vi "detectISOSPIdebug.vi"(8 "errin":errorcluster) -> ()   [LabVIEW 2020]
uses:
  <vilib>/Instr/_visa.llb/VISA Find Search Mode.ctl
  <vilib>/Instr/_visa.llb/VISA Configure Serial Port (Instr).vi
panel:
  out "liste trouvée":string[](array[string])
  out "tableau ajouté":errorcluster[](array[cluster])
  out "Booléen":bool
  out "buffer de lecture":string
  # "2A49 444E 3F0A"
  # "*IDN?"
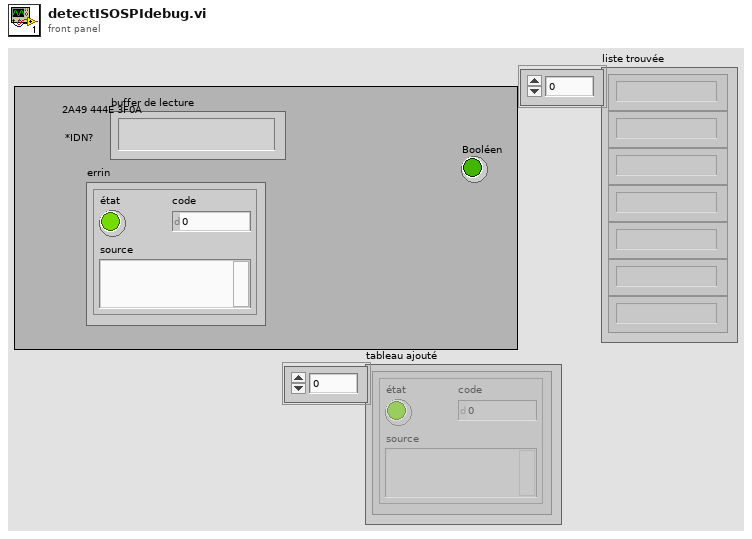
[diagram p1: front panel]
types:
  T1 = typedef "VISA Find Search Mode.ctl" = u32
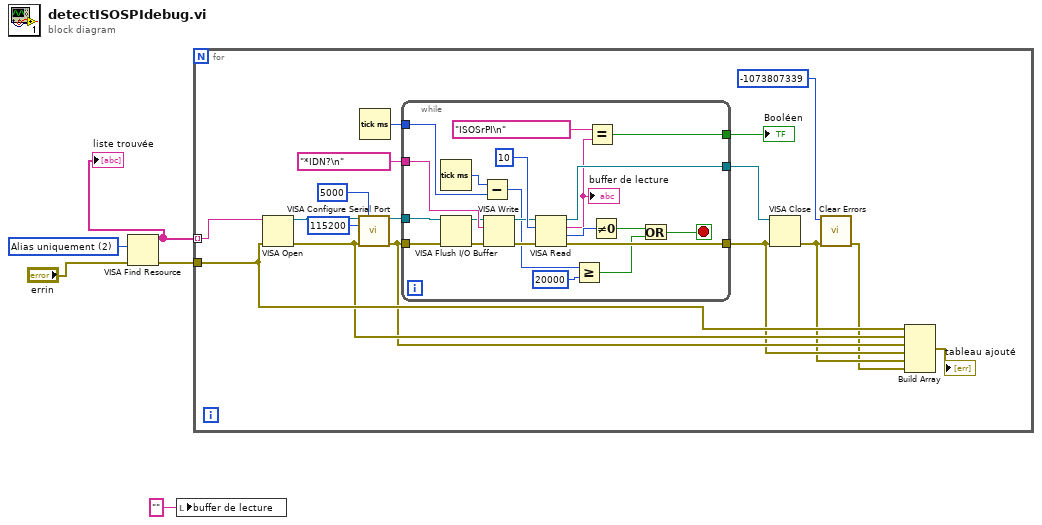
[diagram p0: block diagram]
diagram:
  w4 = T1 2 items=["Noms canoniques uniquement"=0, "Alias uniquement"=2, "Inclure les alias correspondants"=3, "Inclure tous les alias"=4] ("Search Mode")
  n1 = VISA Find Resource(8:"errin", 10:w4) -> (0:w2:errorcluster, 3:w1:string[])  [unwired: 1 in, 1 out]
  "liste trouvée" <- w1
  n2 = local write "buffer de lecture"("" ("buffer de lecture")) -> ()
  n3 = for {
    tunnel: w2 -> [w14]
    tunnel: w1 -> [w7] mode=indexing
    n4 = VISA Open(error in (no error)=w14, VISA resource name=w7) -> (VISA resource name=w21:refnum<visa-resource-name>, error out=w13:errorcluster)  [unwired: 3 in]
    n5 = call-poly "VISA Configure Serial Port"("VISA resource name"=w21, "timeout (10sec)"=u32 5000, "baud rate (9600)"=u32 115200, "error in (no error)"=w13) -> ("VISA resource name out"=w19:refnum<visa-resource-name>, "error out"=w12:errorcluster)  [unwired: 10 in]
    n6 = Tick Count (ms)() -> (millisecond timer value=w22:u32)
    n7 = while {
      tunnel: [w43] -> w11
      tunnel: w12 -> [w35]
      tunnel: "*IDN?\n" ("buffer d'écriture") -> [w40]
      tunnel: w19 -> [w36]
      tunnel: [w38] -> w18
      tunnel: [w30] -> w15
      tunnel: w22 -> [w28]
      stop <- w23 stop-if-true
      n8 = Tick Count (ms)() -> (millisecond timer value=w29:u32)
      n9 = VISA Flush I/O Buffer(VISA resource name=w36, error in (no error)=w35) -> (VISA resource name out=w33:refnum<visa-resource-name>, error out=w34:errorcluster)  [unwired: 1 in]
      n10 = Subtract(x=w29, y=w28) -> (x-y=w27:u32)
      n11 = VISA Write(VISA resource name=w33, write buffer=w40, error in (no error)=w34) -> (VISA resource name out=w37:refnum<visa-resource-name>, error out=w39:errorcluster)  [unwired: 1 out]
      n12 = VISA Read(VISA resource name=w37, byte count=u32 10 ("nombre d'octets"), error in (no error)=w39) -> (VISA resource name out=w38:refnum<visa-resource-name>, read buffer=w32:string, return count=w41:u32, error out=w43:errorcluster)
      "buffer de lecture" <- w32
      n13 = Greater Or Equal? ("Supérieur ou égal ?")(x=w27, y=u32 20000) -> (x >= y?=w25:bool)
      n14 = Equal? ("Égaux ?")(x="ISOSrPI\n", y=w32) -> (x = y?=w30:bool)
      n15 = Not Equal To 0?(x=w41) -> (x != 0?=w24:bool)
      n16 = Or(x=w24, y=w25) -> (x .or. y?=w23:bool)
    }
    "Booléen" <- w15
    n17 = VISA Close(VISA resource name=w18, error in (no error)=w11) -> (error out=w10:errorcluster)
    n18 = call <vilib>:"Clear Errors.vi"("error in (no error)"=w10, "specific error code to clear (0: all)"=-1073807339) -> ("error out"=w9:errorcluster)  [unwired: 4 in, 1 out]
    n19 = Build Array(w14, w13, w12, w11, w10, w9) -> (→"tableau ajouté":errorcluster[])
  }
